vi "Write Laser Configuration.vi"(8 "error in (no error)":errorcluster, 10 "Laser Configuration":T1[](array[typedef]), 11 "Laser Quantum in":refnum<class "Laser Quantum.lvclass">) -> (0 "error out":errorcluster, 3 "Laser Quantum out":refnum<class "Laser Quantum.lvclass">)   [LabVIEW 2015, in "Laser Quantum.lvlib" / "Laser Quantum.lvclass"]
uses:
  Laser Quantum.lvclass
  Resources/Type Defs/Excitation.ctl
  Resources/Type Defs/Laser Configuration.ctl
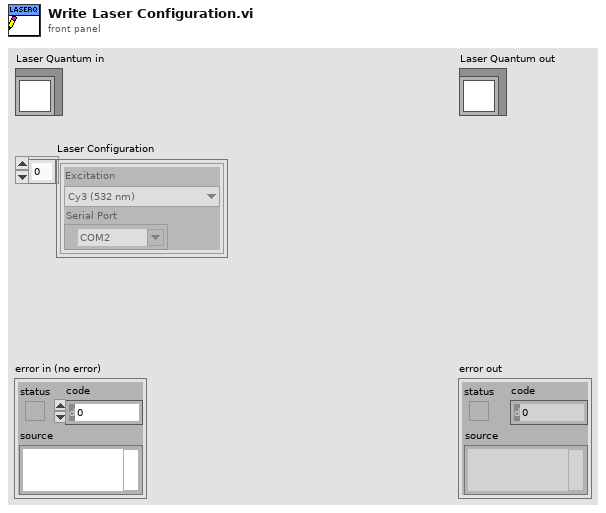
[diagram p1: front panel]
types:
  T1 = typedef "Laser Configuration.ctl" = cluster{"Excitation":T2, "Serial Port":refnum<visa-resource-name>}
  T2 = typedef "Excitation.ctl" = enum16{"Cy2 (473 nm)", "Cy3 (532 nm)", "Cy5 (639 nm)", "Cy7 (730 nm)"}
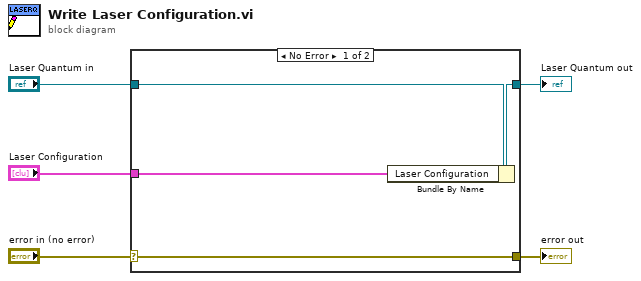
[diagram p0: block diagram]
diagram:
  n1 = case shown="No Error" "error in (no error)" {
    selector: "error in (no error)" -> [w9 w10]
    tunnel: [w9 w10] -> w4
    tunnel: [w7 w11] -> w2
    tunnel: "Laser Quantum in" -> [w8 w11]
    tunnel: "Laser Configuration" -> [w6 _]
    frame No Error {
      n2 = Bundle By Name(cluster=w8, "Laser Configuration"=w6) -> (w7:refnum<class "Laser Quantum.lvclass">)
    }
    frame Error {
    }
  }
  "error out" <- w4
  "Laser Quantum out" <- w2
